vi "Connections to Strings.vi"(8 "error in (no error)":errorcluster, 10 "connection list":T2[](array[typedef]), 11 "Channel Ref in":T1 format="%.0x") -> (0 "error out":errorcluster, 2 "connection strings":string[](array[string]), 3 "Channel Ref out":T1 format="%.0x")   [LabVIEW 2017, in "Routing and Faulting Scripting.lvlib"]
uses:
  Routing and Faulting Scripting.lvlib
  Shared/Connection.ctl
  <vilib>/NI Veristand/Custom Device API/Custom Device Item Ref.ctl
  Shared/Routing and Faulting Shared.lvlib
  <vilib>/NI Veristand/Custom Device API/Custom Device API.lvlib
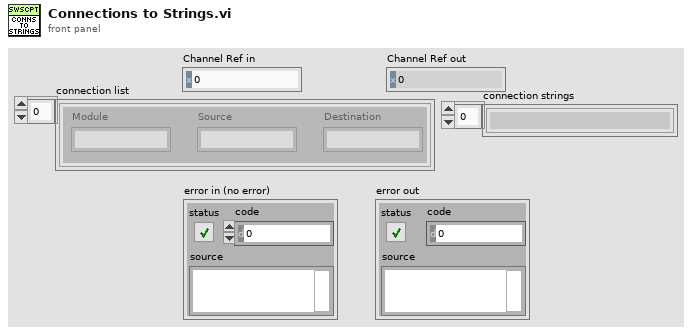
[diagram p1: front panel]
types:
  T1 = typedef "Custom Device API.lvlib/Custom Device Item Ref.ctl" = u64
  T2 = typedef "Routing and Faulting Shared.lvlib/Connection.ctl" = cluster{"Module":string, "Source":string, "Destination":string}
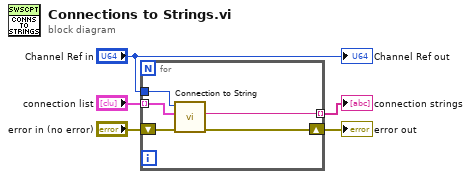
[diagram p0: block diagram]
diagram:
  n1 = for {
    tunnel: "connection list" -> [w10] mode=indexing
    tunnel: [w9] -> w4 mode=indexing
    shift-right: [w7] -> w2
    shift-left: "error in (no error)" -> [w8]
    tunnel: "Channel Ref in" -> [w6]
    n2 = call "Connection to String.vi"("error in (no error)"=w8, "Connection"=w10, "Channel Ref in"=w6) -> ("error out"=w7:errorcluster, "String"=w9:string)  [unwired: 6 in, 1 out]
  }
  "connection strings" <- w4
  "error out" <- w2
  "Channel Ref out" <- "Channel Ref in"
